vi "wait on initialized communicator.vi"(8 "error in":errorcluster, 11 "communicator task in":refnum<class "communicator task.lvclass">) -> (0 "error out":errorcluster, 1 "timed out?":bool, 3 "initialized communicator":refnum<class "communicator.lvclass">)   [LabVIEW 2015, in "communicator task.lvclass"]
uses:
  communicator task.lvclass
  communicator/communicator.lvclass
  communicator task.lvclass/communicator task.ctl
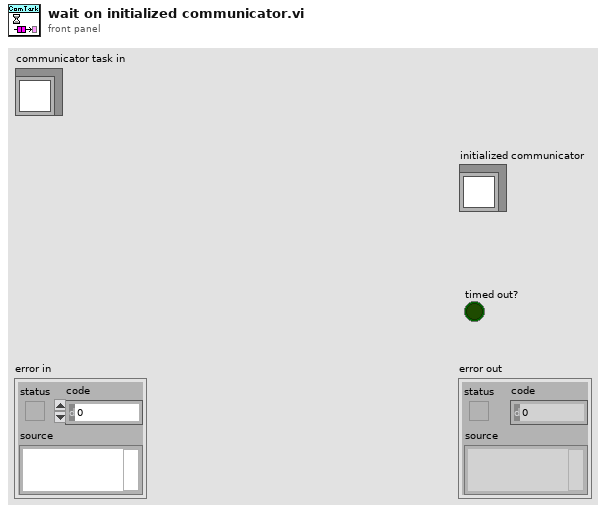
[diagram p1: front panel]
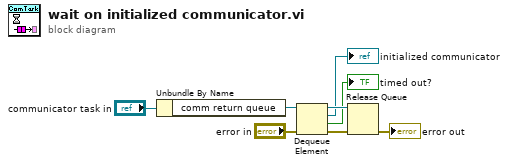
[diagram p0: block diagram]
diagram:
  n1 = Unbundle By Name("communicator task in") -> ("comm return queue"=w2:refnum<queue>)
  n2 = Dequeue Element(queue=w2, error in (no error)="error in") -> (queue out=w7:refnum<queue>, element=→"initialized communicator":refnum<class "communicator.lvclass">, timed out?=→"timed out?":bool, error out=w8:errorcluster)  [unwired: 1 in]
  n3 = Release Queue(queue=w7, error in (no error)=w8) -> (error out=→"error out":errorcluster)  [unwired: 1 in, 2 out]
